vi "test Add-Find-Remove Messages.vi"(8 "error in":errorcluster, 11 "TestCase in":refnum<class "Scripting.lvclass">) -> (0 "error out":errorcluster, 3 "TestCase out":refnum<class "Scripting.lvclass">)   [LabVIEW 2020, in "Scripting.lvclass"]
uses:
  Scripting.lvclass
  C:/dev/git/niveristand-custom-device-testing-tools/VeriStandScriptingTestCase/VeriStandScriptingTestCase.lvclass
  Shared/1553 Channel.ctl
  Shared/Address.ctl
  Shared/Major Frame Definition.ctl
  Shared/Minor Frame Definition.ctl
  Shared/Message Definition.ctl
  Shared/Message Type.ctl
  Shared/Terminal Endpoint.ctl
  Shared/Parameter Definition.ctl
  niveristand-custom-device-testing-tools/VeriStandScriptingTestCase/VeriStandScriptingTestCase.lvclass/VeriStandScriptingTestCase.ctl
  niveristand-custom-device-testing-tools/VeriStandScriptingTestCase/Read Target.vi
  NationalInstruments.VeriStand.SystemDefinitionAPI
  <vilib>/addons/_JKI Toolkits/VI Tester/TestCase.llb/TestCase.lvclass
  Scripting/AIM MIL-STD-1553 Scripting.lvlib
  C:/Program Files (x86)/National Instruments/LabVIEW 2020/vi.lib/addons/_JKI Toolkits/VI Tester/TestCase.llb/TestCase.lvclass
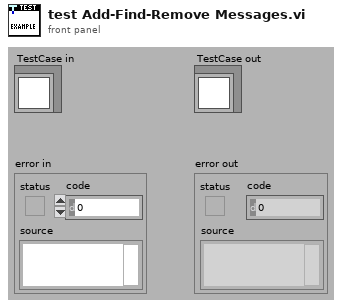
[diagram p1: front panel]
types:
  T1 = typedef "1553 Channel.ctl" = cluster{"HW channel":u16, "terminal addresses":T2[], "terminal names":string[], "acyclic frame names":string[], "major frames":T3[], "minor frames":T4[], "messages":T5[]}
  T2 = typedef "Address.ctl" = u16
  T3 = typedef "Major Frame Definition.ctl" = cluster{"name":string, "minor frames":string[]}
  T4 = typedef "Minor Frame Definition.ctl" = cluster{"name":string, "messages":string[]}
  T5 = typedef "Message Definition.ctl" = cluster{"name":string, "message type":T6, "endpoint Tx":T7, "endpoint Rx":T7, "create timestamp channel":bool, "mode code":u16, "number of words":u16, "parameters":cluster{"name":string, "default value":dbl, "unit":string, "parameter definition":T8}[]}
  T6 = typedef "Message Type.ctl" = string
  T7 = typedef "Terminal Endpoint.ctl" = cluster{"terminal address":T2, "subaddress":T2}
  T8 = typedef "Parameter Definition.ctl" = cluster{"start index":i32, "size (bits)":i32, "encoding":enum16{"BNR", "BCD", "Discrete"}, "signed":bool, "multiplier":dbl, "offset":dbl}
  T9 = typedef "Custom Device API.lvlib/Custom Device Item Ref.ctl" = u64
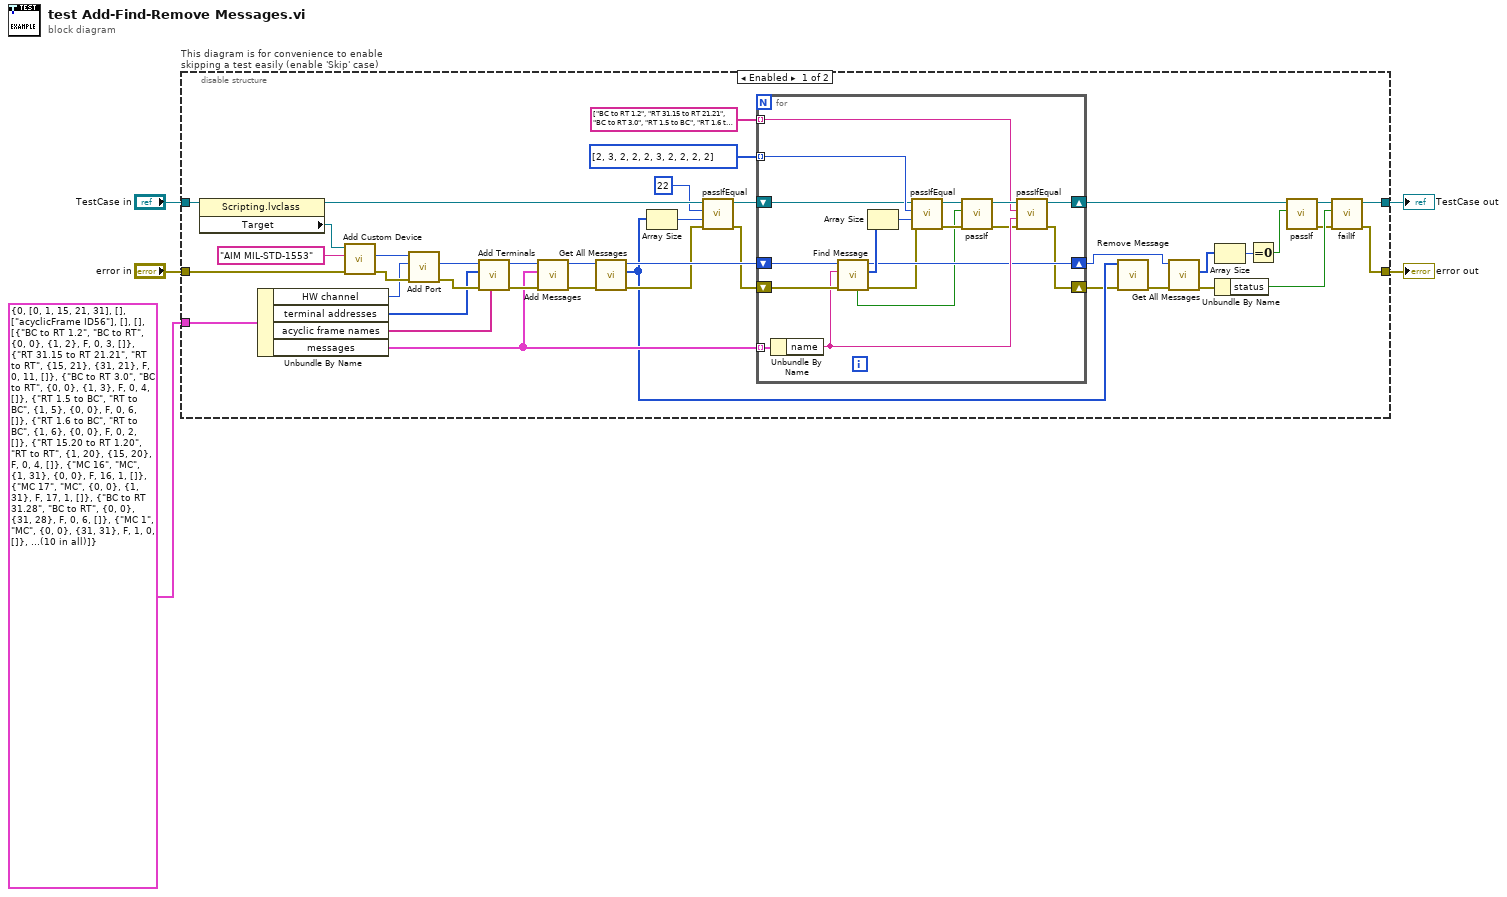
[diagram p0: block diagram]
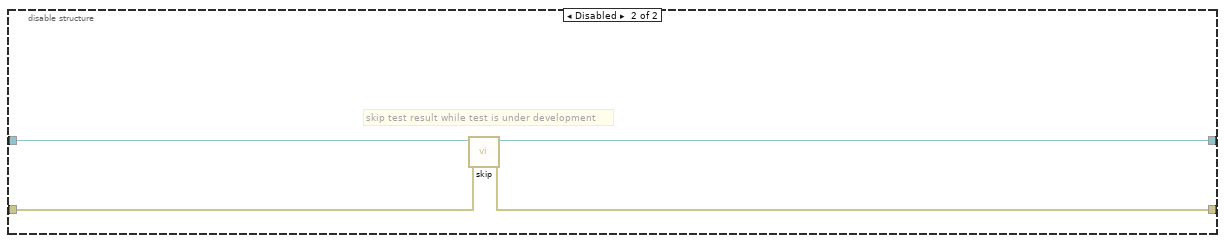
[diagram p2: hidden frame]
diagram:
  n1 = disable-structure "This diagram is for convenience to enable skipping a test easily (enable 'Skip' case)" shown="Enabled" {
    disable-tunnel: "TestCase in" -> [w43 w67]
    disable-tunnel: [w40 w65] -> w2
    disable-tunnel: [w41 w66] -> w4
    disable-tunnel: "error in" -> [w45 w64]
    disable-tunnel: T1 {"HW channel"=0, "terminal addresses"=[0, 1, 15, 21, 31], "terminal names"=[], "acyclic frame names"=["acyclicFrame ID56"], "major frames"=[], "minor frames"=[], "messages"=[{"name"="BC to RT 1.2", "message type"="BC to RT", "endpoint Tx"={"terminal address"=0, "subaddress"=0}, "endpoint Rx"={"terminal address"=1, "subaddress"=2}, "create timestamp channel"=FALSE, "mode code"=0, "number of words"=3, "parameters"=[]}, {"name"="RT 31.15 to RT 21.21", "message type"="RT to RT", "endpoint Tx"={"terminal address"=15, "subaddress"=21}, "endpoint Rx"={"terminal address"=31, "subaddress"=21}, "create timestamp channel"=FALSE, "mode code"=0, "number of words"=11, "parameters"=[]}, {"name"="BC to RT 3.0", "message type"="BC to RT", "endpoint Tx"={"terminal address"=0, "subaddress"=0}, "endpoint Rx"={"terminal address"=1, "subaddress"=3}, "create timestamp channel"=FALSE, "mode code"=0, "number of words"=4, "parameters"=[]}, {"name"="RT 1.5 to BC", "message type"="RT to BC", "endpoint Tx"={"terminal address"=1, "subaddress"=5}, "endpoint Rx"={"terminal address"=0, "subaddress"=0}, "create timestamp channel"=FALSE, "mode code"=0, "number of words"=6, "parameters"=[]}, {"name"="RT 1.6 to BC", "message type"="RT to BC", "endpoint Tx"={"terminal address"=1, "subaddress"=6}, "endpoint Rx"={"terminal address"=0, "subaddress"=0}, "create timestamp channel"=FALSE, "mode code"=0, "number of words"=2, "parameters"=[]}, {"name"="RT 15.20 to RT 1.20", "message type"="RT to RT", "endpoint Tx"={"terminal address"=1, "subaddress"=20}, "endpoint Rx"={"terminal address"=15, "subaddress"=20}, "create timestamp channel"=FALSE, "mode code"=0, "number of words"=4, "parameters"=[]}, {"name"="MC 16", "message type"="MC", "endpoint Tx"={"terminal address"=1, "subaddress"=31}, "endpoint Rx"={"terminal address"=0, "subaddress"=0}, "create timestamp channel"=FALSE, "mode code"=16, "number of words"=1, "parameters"=[]}, {"name"="MC 17", "message type"="MC", "endpoint Tx"={"terminal address"=0, "subaddress"=0}, "endpoint Rx"={"terminal address"=1, "subaddress"=31}, "create timestamp channel"=FALSE, "mode code"=17, "number of words"=1, "parameters"=[]}, {"name"="BC to RT 31.28", "message type"="BC to RT", "endpoint Tx"={"terminal address"=0, "subaddress"=0}, "endpoint Rx"={"terminal address"=31, "subaddress"=28}, "create timestamp channel"=FALSE, "mode code"=0, "number of words"=6, "parameters"=[]}, {"name"="MC 1", "message type"="MC", "endpoint Tx"={"terminal address"=0, "subaddress"=0}, "endpoint Rx"={"terminal address"=31, "subaddress"=31}, "create timestamp channel"=FALSE, "mode code"=1, "number of words"=0, "parameters"=[]}]} ("1553 channel") -> [w6 _]
    frame Enabled {
      n2 = property class="Scripting.lvclass"(reference=w43) -> (reference out=w27:refnum<class "Scripting.lvclass">, "Target"=w42:refnum<k24>)  [unwired: 1 in, 1 out]
      n3 = Unbundle By Name(w6) -> ("HW channel"=w35:u16, "terminal addresses"=w30:T2[], "acyclic frame names"=w29:string[], "messages"=w24:T5[])
      n4 = call "Add Custom Device.vi"("error in"=w45, "custom device name"="AIM MIL-STD-1553" ("name"), "target"=w42) -> ("error out"=w38:errorcluster, "custom device ref out"=w37:T9)  [unwired: 6 in, 1 out]
      n5 = call "Add Port.vi"("error in"=w38, "port number"=w35, "custom device ref"=w37) -> ("error out"=w33:errorcluster, "port"=w34:T9)  [unwired: 6 in, 1 out]
      n6 = call "Add Terminals.vi"("acyclic frame names"=w29, "error in"=w33, "terminal addresses"=w30, "port in"=w34) -> ("error out"=w31:errorcluster, "port out"=w32:T9)  [unwired: 6 in]
      n7 = call "Add Messages.vi"("error in"=w31, "messages"=w24, "port in"=w32) -> ("error out"=w28:errorcluster, "port out"=w36:T9)  [unwired: 7 in]
      n8 = call "Get All Messages.vi"("error in"=w28, "port in"=w36) -> ("error out"=w22:errorcluster, "messages"=w20:T9[], "port out"=w25:T9)  [unwired: 7 in]
      n9 = Array Size(array=w20) -> (size(s)=w26:i32)
      n10 = call-dynamic "passIfEqual.vi"("error in (no error)"=w22, "y"=w26, "x"=22 ("size(s)"), "TestCase in"=w27) -> ("error out"=w21:errorcluster, "TestCase out"=w8:refnum<class "Scripting.lvclass">)  [unwired: 6 in]
      n11 = for {
        shift-right: [w47] -> w7
        shift-left: w21 -> [w62]
        tunnel: w24 -> [w61] mode=indexing
        shift-right: [w58] -> w17
        shift-left: w25 -> [w63]
        tunnel: string[] ["BC to RT 1.2", "RT 31.15 to RT 21.21", "BC to RT 3.0", "RT 1.5 to BC", "RT 1.6 to BC", "RT 15.20 to RT 1.20", "MC 16", "MC 17", "BC to RT 31.28", "MC 1"] ("Array") -> [w53] mode=indexing
        tunnel: i32[] [2, 3, 2, 2, 2, 3, 2, 2, 2, 2] ("Array 3") -> [w52] mode=indexing
        shift-right: [w51] -> w9
        shift-left: w8 -> [w49]
        n12 = Unbundle By Name(w61) -> ("name"=w60:string)
        n13 = call "Find Message.vi"("error in"=w62, "message name"=w60, "port in"=w63) -> ("error out"=w48:errorcluster, "message refs"=w59:T9[], "port out"=w58:T9, "found?"=w46:bool)  [unwired: 5 in]
        n14 = Array Size(array=w59) -> (size(s)=w50:i32)
        n15 = call-dynamic "passIfEqual.vi"("error in (no error)"=w48, "y"=w50, "x"=w52, "TestCase in"=w49) -> ("error out"=w55:errorcluster, "TestCase out"=w54:refnum<class "Scripting.lvclass">)  [unwired: 6 in]
        n16 = call-dynamic "passIf.vi"("error in (no error)"=w55, "pass"=w46, "TestCase in"=w54) -> ("error out"=w57:errorcluster, "TestCase out"=w56:refnum<class "Scripting.lvclass">)  [unwired: 7 in]
        n17 = call-dynamic "passIfEqual.vi"("error in (no error)"=w57, "y"=w60, "x"=w53, "TestCase in"=w56) -> ("error out"=w47:errorcluster, "TestCase out"=w51:refnum<class "Scripting.lvclass">)  [unwired: 6 in]
      }
      n18 = call "Remove Message.vi"("error in"=w7, "message refs"=w20) -> ("error out"=w19:errorcluster)  [unwired: 9 in]
      n19 = call "Get All Messages.vi"("error in"=w19, "port in"=w17) -> ("error out"=w18:errorcluster, "messages"=w16:T9[])  [unwired: 7 in, 1 out]
      n20 = Array Size(array=w16) -> (size(s)=w15:i32)
      n21 = Unbundle By Name(w18) -> ("status"=w39:bool)
      n22 = Equal To 0?(x=w15) -> (x = 0?=w14:bool)
      n23 = call-dynamic "passIf.vi"("pass"=w14, "TestCase in"=w9) -> ("error out"=w12:errorcluster, "TestCase out"=w13:refnum<class "Scripting.lvclass">)  [unwired: 8 in]
      n24 = call-dynamic "failIf.vi"("error in (no error)"=w12, "fail"=w39, "TestCase in"=w13) -> ("error out"=w41:errorcluster, "TestCase out"=w40:refnum<class "Scripting.lvclass">)  [unwired: 7 in]
    }
    frame Disabled {
      # "skip test result while test is under development"
      n25 = call <vilib>:"skip.vi"("error in (no error)"=w64, "TestCase in"=w67) -> ("error out"=w66:errorcluster, "TestCase out"=w65:refnum<class "Scripting.lvclass">)  [unwired: 8 in]
    }
  }
  "error out" <- w4
  "TestCase out" <- w2
